vi "Dialog_Update Settings Information.vi"(8 "error in (no error)":errorcluster, 11 "Setting File Type":T2=enum."Configuration Settings") -> (0 "error out":errorcluster)   [LabVIEW 2012]
doc: "SciScan 1.2 160622"
uses:
  Custom Controls/Setting File Types.ctl
  SubVIs/FGV_Macro Settings to GFG_Command.ctl
  Custom Controls and Typedefs/GFG Variable for IO.ctl
panel:
  in  "Advanced View?":bool
  out "Array":T1(array[cluster])
  out "Message String":string
  # "You are currently in SciScript Edit Mode. Use SciScan main user interface to adjust scan settings, then press 'Confirm' (blinking) in SciScript module to save settings. (n.b: To ensure that you record from the desired XYZ position it is strongly recommended to add a Move.To.Position action in the line above each scan.)"
  # "Select 'Cancel' (in SciScript module) to abort."
  # "GFG Variable Name"
  # "Value"
  # "Data Type"
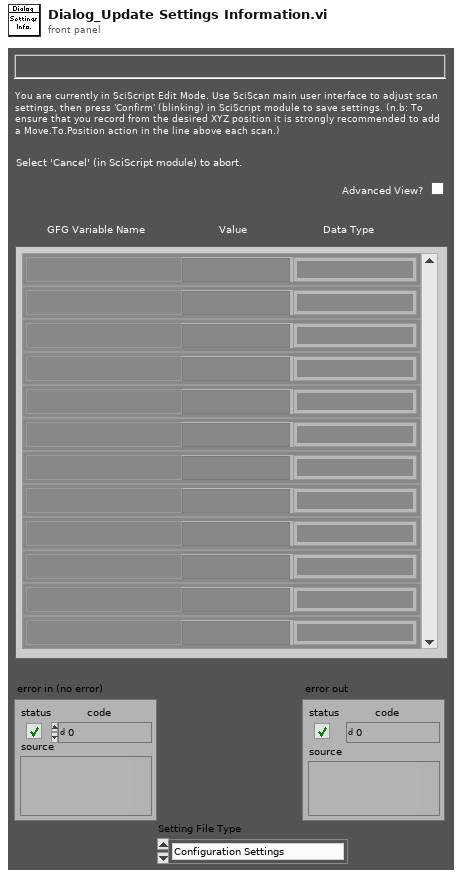
[diagram p1: front panel]
types:
  T1 = cluster{"Name":string, "Variant":variant, "Type":string}[]
  T2 = typedef "Setting File Types.ctl" = enum16{"2D.Frame.Scan.Settings", "2D.Line.Scan.Settings", "Z.Stack.Settings", "HW Settings", "Configuration Settings", "Unknown Settings", "Fast.Z.Settings"}
  T3 = typedef "FGV_Macro Settings to GFG_Command.ctl" = enum16{"Get Current Settings", "Backup Curent Settings", "Recover Backed up settings", "Overwrite Current Settings"}
  T4 = typedef "LVRectTypeDef.ctl" = cluster{"Left":i16, "Top":i16, "Right":i16, "Bottom":i16}
  T5 = typedef "GFG Variable for IO.ctl" = cluster{"Variable Name":string, "Value (Variant)":variant, "data type":string}
  T6 = typedef "VariantType.lvlib/Type.ctl" = enum8{"Invalid Type", "Void", "I8", "I16", "I32", "I64", "U8", "U16", "U32", "U64", "Single Float", "Double Float", "Extended Float", "Single Complex", "Double Complex", "Extended Complex", "Enum U8", "Enum U16", "Enum U32", "Enum U64", "Single Float With Unit", "Double Float With Unit", "Extended Float With Unit", "Single Complex with Unit", "Double Complex with Unit", "Extended Complex with Unit", "Boolean", "String", "Path", "Picture", "Tag", "Array", "Cluster", "Variant", "LV Variant", "Waveform", "Timestamp", "Digital Waveform", "Digital Data", "ExpressData", "Refnum", "External Data", "VI", "Poly VI", "LabVIEW Class Instance", "Fixed Point"}
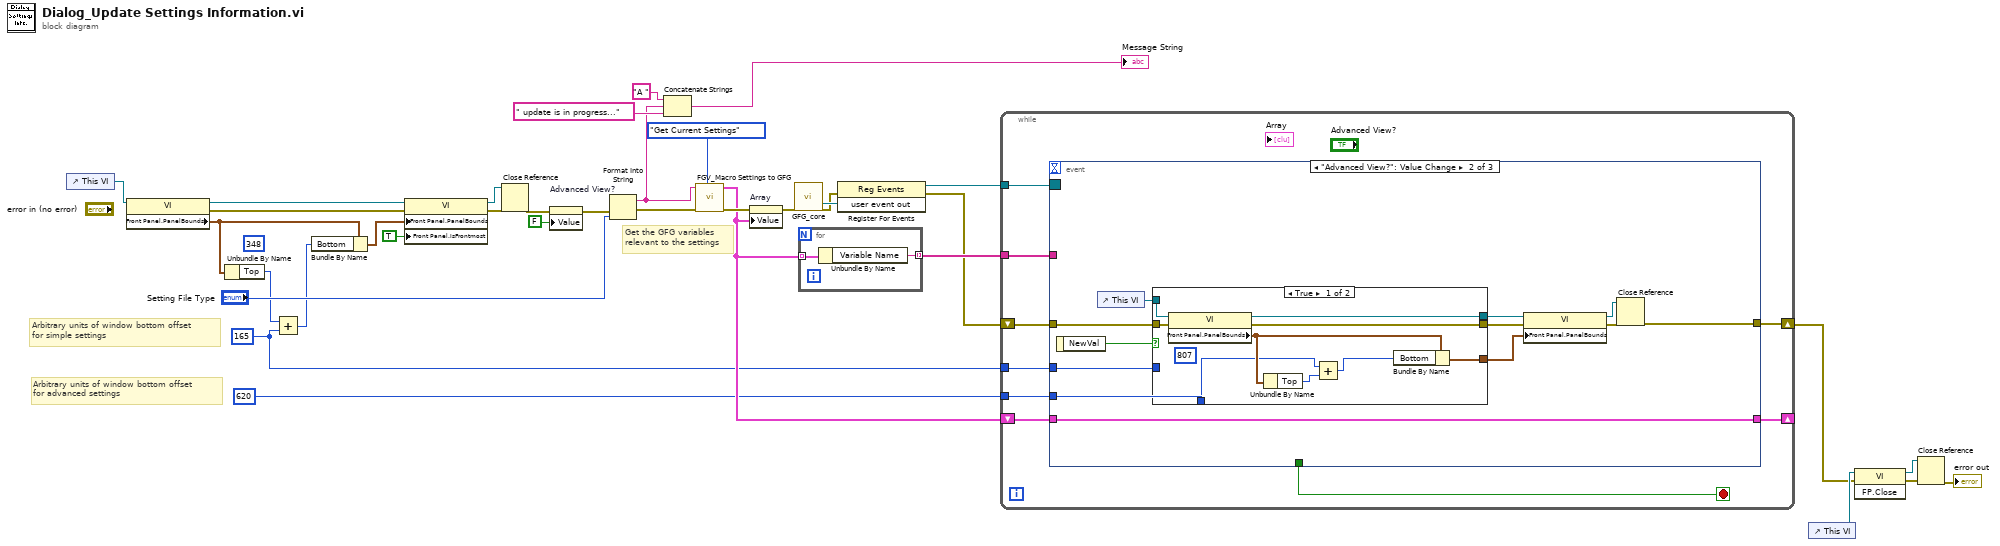
[diagram p0: block diagram]
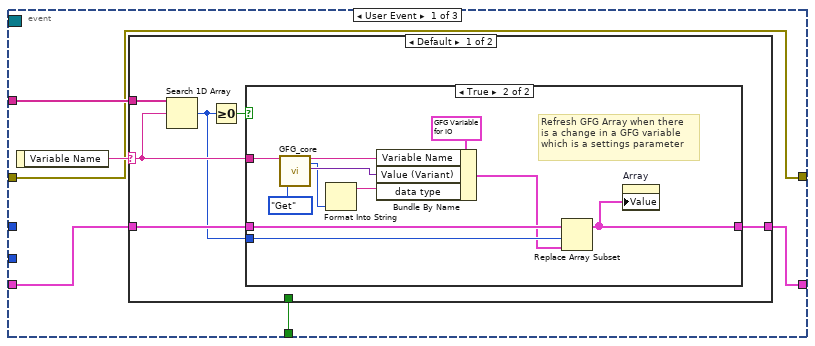
[diagram p2: hidden frame]
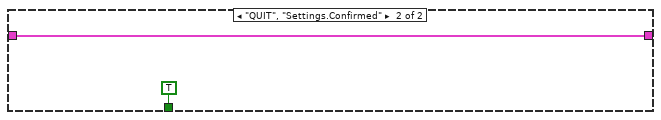
[diagram p4: hidden frame]
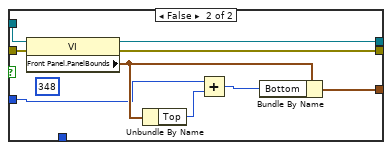
[diagram p5: hidden frame]
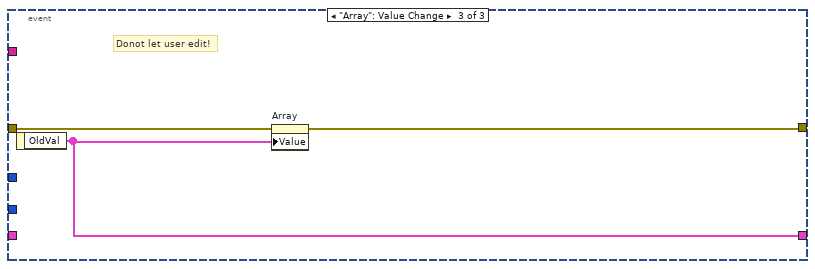
[diagram p6: hidden frame]
diagram:
  w2 = i16 165 ("y")
  (unwired) i16 348 ("Bottom")
  # "Arbitrary units of window bottom offset\nfor simple settings"
  # "Arbitrary units of window bottom offset\nfor advanced settings"
  # "Get the GFG variables\nrelevant to the settings"
  n1 = control-ref of="This VI"() -> (w12:refnum<vi>)
  n2 = property class="VI"(reference=w12) -> (reference out=w14:refnum<vi>, error out=w15:errorcluster, "Front Panel.PanelBounds"=w5:T4)  [unwired: 1 in]
  n3 = Unbundle By Name(w5) -> ("Top"=w4:i16)
  n4 = Add(x=w4, y=w2) -> (x+y=w3:i16)
  n5 = Bundle By Name(cluster=w5, "Bottom"=w3) -> (w13:T4)
  n6 = property class="VI"(reference=w14, error in=w15, "Front Panel.PanelBounds"=w13, "Front Panel.IsFrontmost"=TRUE ("Front Panel Window:Is Frontmost")) -> (reference out=w9:refnum<vi>, error out=w10:errorcluster)
  n7 = Close Reference(reference=w9, error in (no error)=w10) -> (error out=w8:errorcluster)
  n8 = property on="Advanced View?" class="Bool (strict)"(error in=w8, "Value"=FALSE ("Advanced View?")) -> (error out=w7:errorcluster)  [unwired: 1 in, 1 out]
  n9 = Format Into String(error in=w7, "Setting File Type") -> (resulting string=w30:string, error out=w16:errorcluster)  [unwired: 2 in]
  n10 = Concatenate Strings("A " ("resulting string"), w30, " update is in progress..." ("string")) -> (→"Message String":string)
  n11 = call "FGV_Macro Settings to GFG.vi"("FGV_Macro Settings to GFG_Command"=FGV_Macro_Settings_to_GFG_Command."Get Current Settings", "error in (no error)"=w16, "Settings type string IN"=w30) -> ("error out"=w29:errorcluster, "Current Settings OUT"=w23:T5[])  [unwired: 6 in, 1 out]
  n12 = property on="Array" class="Arr (strict)"(error in=w29, "Value"=w23) -> (error out=w26:errorcluster)  [unwired: 1 in, 1 out]
  n13 = call "GFG_core.vi"("error in (no error)"=w26) -> ("user event out"=w28:refnum<user-event>, "error out"=w27:errorcluster)  [unwired: 12 in, 5 out]
  n14 = for {
    tunnel: w23 -> [w37] mode=indexing
    tunnel: [w36] -> w24 mode=indexing
    n15 = Unbundle By Name(w37) -> ("Variable Name"=w36:string)
  }
  n16 = register-events(error in=w27, w28) -> (reference out=w25:refnum<event-registration>, error out=w22:errorcluster)  [unwired: 1 in]
  n17 = while {
    tunnel: w25 -> [w45]
    tunnel: w24 -> [w44]
    shift-right: [w43] -> _
    shift-left: w23 -> [w42]
    shift-right: [w40] -> w20
    shift-left: w22 -> [w41]
    tunnel: i16 620 ("y") -> [w39]
    tunnel: w2 -> [w38]
    stop <- w46 stop-if-true
    n18 = event shown="[1] \"Advanced View?\": Value Change" {
      selector: w45 -> [_ _ _]
      dyn-events: _ -> [_ _ _]
      timeout: _ -> [_ _ _]
      tunnel: [w51 _ _] -> w46
      tunnel: w44 -> [w50 _ _]
      tunnel: [w49 w84 w105] -> w43
      tunnel: w42 -> [w48 w84 _]
      tunnel: w41 -> [w47 w81 w104]
      tunnel: [w47 w75 w103] -> w40
      tunnel: w39 -> [_ w74 _]
      tunnel: w38 -> [_ w73 _]
      event User Event {
        n19 = event-data() -> ("Variable Name"=w52:string)  [unwired: 1 in]
        n20 = case shown="Default" w52 {
          selector: w52 -> [w56 _]
          tunnel: [_ TRUE] -> w51
          tunnel: w50 -> [w58 _]
          tunnel: [w55 w71] -> w49
          tunnel: w48 -> [w54 w71]
          frame Default {
            n21 = Search 1D Array(1D array=w58, element=w56) -> (index of element=w53:i32)  [unwired: 1 in]
            n22 = Greater Or Equal To 0?(x=w53) -> (x >= 0?=w57:bool)
            n23 = case shown="True" w57 {
              tunnel: w56 -> [_ w69]
              tunnel: [w59 w60] -> w55
              tunnel: w54 -> [w59 w68]
              tunnel: w53 -> [_ w67]
              frame False {
              }
              frame True {
                # "Refresh GFG Array when there\nis a change in a GFG variable \nwhich is a settings parameter"
                n24 = call "GFG_core.vi"("Variable Name in"=w69, "Action"=enum16{"Init", "Set", "Get", "Clear"}."Get") -> ("Variable Name Out"=w64:string, "Data Type Out"=w63:T6, "Variant Out"=w65:variant)  [unwired: 11 in, 4 out]
                n25 = Format Into String(w63) -> (resulting string=w62:string)  [unwired: 3 in, 1 out]
                n26 = Bundle By Name(cluster=T5 {"Variable Name"="", "Value (Variant)"=variant, "data type"=""} ("GFG Vairable for IO"), "Variable Name"=w64, "Value (Variant)"=w65, "data type"=w62) -> (w61:T5)
                n27 = Replace Array Subset(array=w68, new element=w61, index=w67) -> (w60:T5[])
                n28 = property on="Array" class="Arr (strict)"("Value"=w60) -> ()  [unwired: 2 in, 2 out]
              }
            }
          }
          frame "QUIT", "Settings.Confirmed" {
          }
        }
      }
      event "Advanced View?": Value Change {
        n29 = event-data() -> ("NewVal"=w83:bool)  [unwired: 1 in]
        n30 = control-ref of="This VI"() -> (w82:refnum<vi>)
        n31 = case shown="True" w83 {
          tunnel: w82 -> [w93 w102]
          tunnel: w81 -> [w92 w101]
          tunnel: [w91 w100] -> w80
          tunnel: [w90 w99] -> w79
          tunnel: [w89 w98] -> w78
          tunnel: w74 -> [w86 _]
          tunnel: w73 -> [_ w95]
          frame True {
            (unwired) i16 807 ("Bottom")
            n32 = property class="VI"(reference=w93, error in=w92) -> (reference out=w90:refnum<vi>, error out=w89:errorcluster, "Front Panel.PanelBounds"=w88:T4)
            n33 = Unbundle By Name(w88) -> ("Top"=w87:i16)
            n34 = Add(x=w86, y=w87) -> (x+y=w85:i16)
            n35 = Bundle By Name(cluster=w88, "Bottom"=w85) -> (w91:T4)
          }
          frame False {
            (unwired) i16 348 ("Bottom")
            n36 = property class="VI"(reference=w102, error in=w101) -> (reference out=w99:refnum<vi>, error out=w98:errorcluster, "Front Panel.PanelBounds"=w97:T4)
            n37 = Unbundle By Name(w97) -> ("Top"=w96:i16)
            n38 = Add(x=w95, y=w96) -> (x+y=w94:i16)
            n39 = Bundle By Name(cluster=w97, "Bottom"=w94) -> (w100:T4)
          }
        }
        n40 = property class="VI"(reference=w79, error in=w78, "Front Panel.PanelBounds"=w80) -> (reference out=w76:refnum<vi>, error out=w77:errorcluster)
        n41 = Close Reference(reference=w76, error in (no error)=w77) -> (error out=w75:errorcluster)
      }
      event "Array": Value Change {
        # "Donot let user edit!"
        n42 = event-data() -> ("OldVal"=w105:T1)  [unwired: 1 in]
        n43 = property on="Array" class="Arr (strict)"(error in=w104, "Value"=w105) -> (error out=w103:errorcluster)  [unwired: 1 in, 1 out]
      }
    }
  }
  n44 = control-ref of="This VI"() -> (w21:refnum<vi>)
  n45 = invoke class="VI" method="FP.Close"(reference=w21, error in=w20) -> (reference out=w18:refnum<vi>, error out=w19:errorcluster)  [unwired: 1 in, 1 out]
  n46 = Close Reference(reference=w18, error in (no error)=w19) -> (error out=→"error out":errorcluster)
